vi "Open unZipSelect File-b.vi"(4 "error in (no error)":errorcluster, 7 "target":path) -> (0 "error out":errorcluster, 3 "unzip file out":i64)   [LabVIEW 2024]
doc: "Creates a new empty zip file in the path that <B>target</B> specifies. The new file overwrites an existing file or produces a confirmation dialog based on the value of the <B>confirm overwrite?</B> control."
panel:
  in  "open":string="Error opening the zip file."
  in  "empty":string="Empty zip file path."
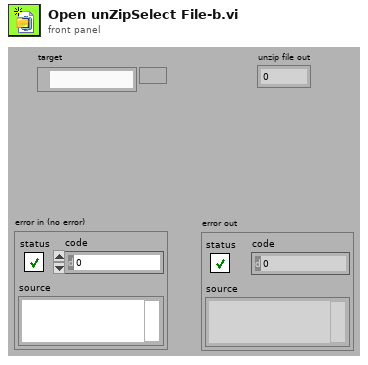
[diagram p1: front panel]
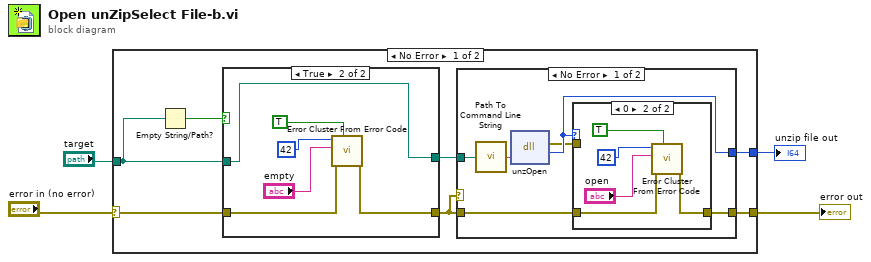
[diagram p0: block diagram]
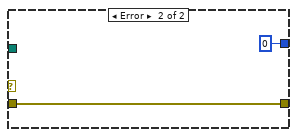
[diagram p3: hidden frame]
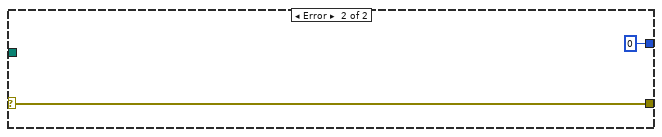
[diagram p5: hidden frame]
diagram:
  n1 = case shown="No Error" "error in (no error)" {
    selector: "error in (no error)" -> [w7 w35]
    tunnel: "target" -> [w5 _]
    tunnel: [w10 w35] -> w1
    tunnel: [w9 i64 0] -> w3
    frame No Error {
      n2 = Empty String/Path?(string/path=w5) -> (empty?=w6:bool)
      n3 = case shown="True" w6 {
        tunnel: w5 -> [w27 w31]
        tunnel: [w27 w31] -> w11
        tunnel: w7 -> [w26 w33]
        tunnel: [w26 w32] -> w8
        frame False {
        }
        frame True {
          n4 = call <vilib>:"Error Cluster From Error Code.vi"("show call chain? (False)"=TRUE ("status"), "error in (no error)"=w33, "error message (\"\")"="empty", "error code (0)"=42 ("code")) -> ("error out"=w32:errorcluster)  [unwired: 5 out]
        }
      }
      n5 = case shown="No Error" w8 {
        tunnel: w11 -> [w16 _]
        tunnel: [w15 w25] -> w10
        tunnel: [w14 i64 0] -> w9
        tunnel: w8 -> [w13 w25]
        frame No Error {
          n6 = call <vilib>:"Path To Command Line String.vi"("path"=w16) -> ("string"=w17:string)
          n7 = dll-call lib="LabVIEW" fn="unzOpen" label="zipOpen"("pathname"=w17) -> (error out=w12:errorcluster, "return type"=w14:i64)  [unwired: 4 in, 1 out]
          n8 = case shown="0" w14 {
            tunnel: [w18 w20] -> w15
            tunnel: w13 -> [w18 w21]
            tunnel: w12 -> [_ _]
            frame Default {
            }
            frame 0 {
              n9 = call <vilib>:"Error Cluster From Error Code.vi"("show call chain? (False)"=TRUE ("status"), "error in (no error)"=w21, "error message (\"\")"="open", "error code (0)"=42 ("code")) -> ("error out"=w20:errorcluster)  [unwired: 5 out]
            }
          }
        }
        frame Error {
        }
      }
    }
    frame Error {
    }
  }
  "unzip file out" <- w3
  "error out" <- w1
